vi "Process Data Buffer, Mode 1.vi"(0 "DATA_Buffer excluding '#' [1...N]":string, 1 "P constants":T1[](array[typedef])) -> (2 "Pressures (Pa)":sgl[](array[numeric]), 3 "Sensor temps (degC)":sgl[](array[numeric]), 4 "Statuses":u8[](array[numeric]), 5 "dt_warn":u8)   [LabVIEW 2020]
uses:
  Ctls/Pressure sensor constants.ctl
panel:
  # "0: valid data\n1: cmd mode\n2: stale data\n3: diag mode"
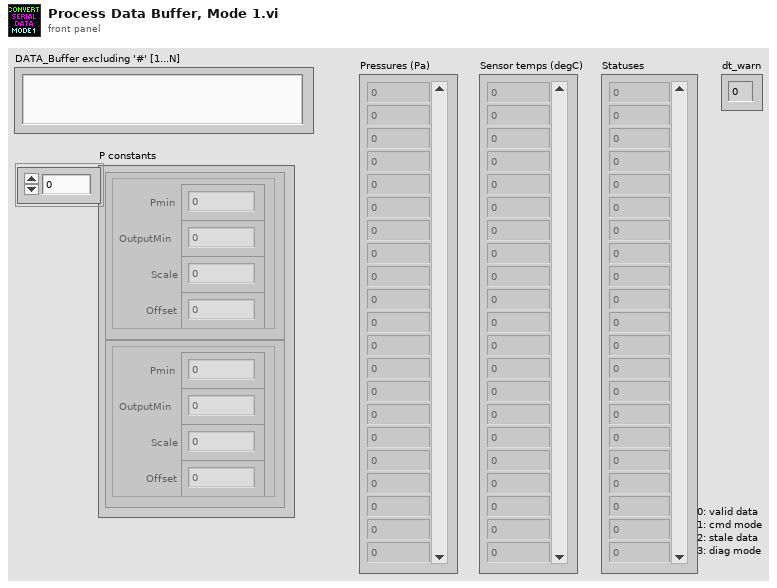
[diagram p1: front panel]
types:
  T1 = typedef "Pressure sensor constants.ctl" = cluster{"Pmin":sgl, "OutputMin":sgl, "Scale":sgl, "Offset":sgl}
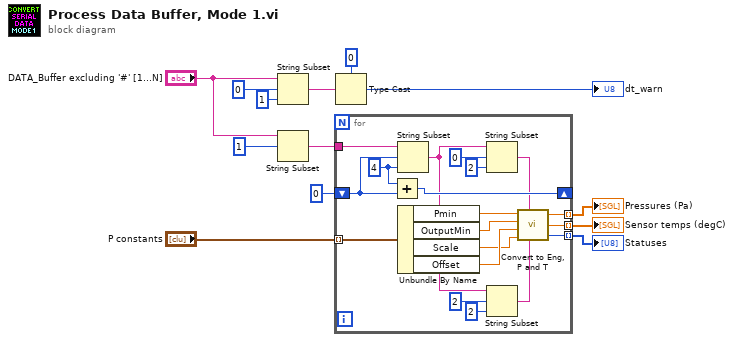
[diagram p0: block diagram]
diagram:
  n1 = String Subset(string="DATA_Buffer excluding '#' [1...N]", offset (0)=0, length (rest)=1 ("length (rest)")) -> (substring=w11:string)
  n2 = String Subset(string="DATA_Buffer excluding '#' [1...N]", offset (0)=1) -> (substring=w6:string)  [unwired: 1 in]
  n3 = for {
    tunnel: w6 -> [w30]
    tunnel: [w32] -> w3 mode=indexing
    tunnel: [w31] -> w2 mode=indexing
    shift-right: [w28] -> _
    shift-left: 0 ("offset (0)") -> [w27]
    tunnel: "P constants" -> [w26] mode=indexing
    tunnel: [w21] -> w1 mode=indexing
    w29 = 4 ("length (rest)")
    n4 = Add(x=w29, y=w27) -> (x+y=w28:i32)
    n5 = String Subset(string=w30, offset (0)=w27, length (rest)=w29) -> (substring=w15:string)
    n6 = Unbundle By Name(w26) -> ("Pmin"=w25:sgl, "OutputMin"=w24:sgl, "Scale"=w22:sgl, "Offset"=w23:sgl)
    n7 = String Subset(string=w15, offset (0)=0, length (rest)=2 ("length (rest)")) -> (substring=w18:string)
    n8 = String Subset(string=w15, offset (0)=2, length (rest)=2 ("length (rest)")) -> (substring=w16:string)
    n9 = call "Convert to Eng, P and T.vi"("Pmin (Pa)"=w25, "P word"=w18, "OutputMin (counts)"=w24, "Poffset (Pa)"=w23, "T word"=w16, "(Pmax - Pmin) / (OutputMax - OutputMin) (Pa/count)"=w22) -> ("P (Pa)"=w32:sgl, "T (degC)"=w21:sgl, "Status bit"=w31:u8)
  }
  "Pressures (Pa)" <- w3
  "Statuses" <- w2
  "Sensor temps (degC)" <- w1
  n10 = Type Cast(type=u8 0, x=w11) -> (*(type *) &x=→"dt_warn":u8)
